vi "Read_Data.vi"(8 "error in":errorcluster caption="entrée d'erreur") -> (0 "error out":errorcluster caption="sortie d'erreur", 1 "AO Slave":waveform(dbl)[](array[waveform]), 2 "AO Master":waveform(dbl)[](array[waveform]), 3 "DO Master":digitalwaveform(graph))   [LabVIEW 2026]
panel:
  out "nom des voies en sortie 3":string[](array[string])
  out "nom des voies en sortie 2":string[](array[string])
  out "nom des voies en sortie":string[](array[string])
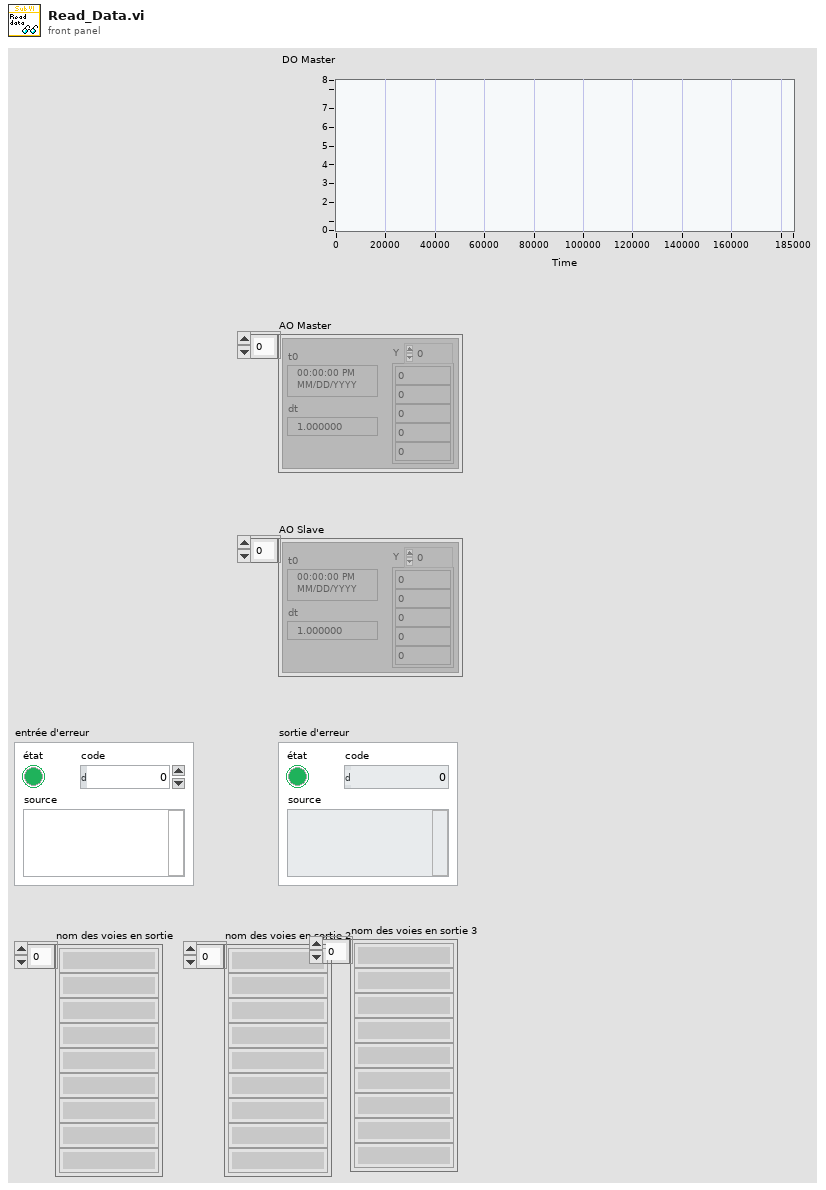
[diagram p1: front panel]
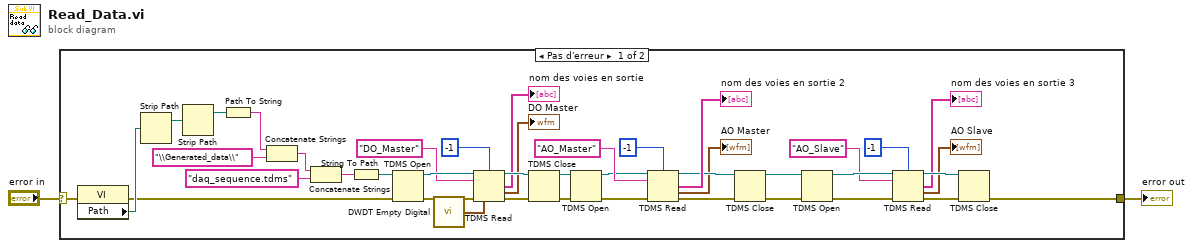
[diagram p0: block diagram]
diagram:
  n1 = case shown="Pas d'erreur" "error in" {
    selector: "error in" -> [w36 w44]
    tunnel: [w4 w44] -> w1
    frame No Error {
      n2 = property class="VI"(error in=w36) -> (error out=w31:errorcluster, "Path"=w42:path)  [unwired: 1 in, 1 out]
      n3 = Strip Path(path=w42) -> (stripped path=w41:path)  [unwired: 1 out]
      n4 = Strip Path(path=w41) -> (stripped path=w40:path)  [unwired: 1 out]
      n5 = Path To String(path=w40) -> (string=w43:string)
      n6 = Concatenate Strings(w43, "\\Generated_data\\" ("Python_file")) -> (w37:string)
      n7 = Concatenate Strings(w37, "daq_sequence.tdms" ("File_to_read")) -> (w32:string)
      n8 = String To Path(string=w32) -> (path=w16:path)
      n9 = TDMS Open(8:w31, 11:w16) -> (0:w33:errorcluster, 3:w30:refnum<k34>)  [unwired: 5 in]
      n10 = call <vilib>:"DWDT Empty Digital.vi"() -> ("digital waveform out"=w26:digitalwaveform)  [unwired: 5 in]
      n11 = TDMS Read(0:w30, 2:i64 -1 ("nombre (-1: tous)"), 5:"DO_Master" ("nom du groupe en entrée"), 11:w33, 12:w26) -> (4:w35:refnum<k34>, 8:→"nom des voies en sortie":string[], 10:→"DO Master":digitalwaveform, 15:w34:errorcluster)  [unwired: 3 in, 2 out]
      n12 = TDMS Close(8:w34, 11:w35) -> (0:w17:errorcluster, 3:w15:path)
      n13 = TDMS Open(8:w17, 11:w15) -> (0:w20:errorcluster, 3:w21:refnum<k34>)  [unwired: 5 in]
      n14 = TDMS Read(0:w21, 2:i64 -1 ("nombre (-1: tous)"), 5:"AO_Master" ("nom du groupe en entrée"), 11:w20) -> (4:w18:refnum<k34>, 8:→"nom des voies en sortie 2":string[], 10:→"AO Master":waveform(dbl)[], 15:w19:errorcluster)  [unwired: 4 in, 2 out]
      n15 = TDMS Close(8:w19, 11:w18) -> (0:w6:errorcluster, 3:w7:path)
      n16 = TDMS Open(8:w6, 11:w7) -> (0:w12:errorcluster, 3:w11:refnum<k34>)  [unwired: 5 in]
      n17 = TDMS Read(0:w11, 2:i64 -1 ("nombre (-1: tous)"), 5:"AO_Slave" ("nom du groupe en entrée"), 11:w12) -> (4:w14:refnum<k34>, 8:→"nom des voies en sortie 3":string[], 10:→"AO Slave":waveform(dbl)[], 15:w13:errorcluster)  [unwired: 4 in, 2 out]
      n18 = TDMS Close(8:w13, 11:w14) -> (0:w4:errorcluster)  [unwired: 1 out]
    }
    frame Error {
    }
  }
  "error out" <- w1
